vi "RubikStart.vi"() -> (0 "error out":errorcluster)   [LabVIEW 2017, in "RubikLibraryRT.lvlib"]
doc: "Put Rubik's solver into start positions:\nAll servos to 0°, all grippers to closed. \nYou have to position the cube manually!\n\nInput:\n-\n\nOutput:\nError out"
uses:
  RubikLibraryRT.lvlib
  ServoEnumControl.ctl
  ServoAbsAngleControl.ctl
  <vilib>/ErrorRing/Error Ring.xnode
  RubikLibrary.lvlib
panel:
  in  "List of Servo Angles":T1[](array[typedef])=[enum."0°", enum."0°", enum."0°"]
  in  "Gripper closed":bool=TRUE
  in  "List of Servos":T2[](array[typedef])=[enum."Left Servo", enum."Front Servo", enum."Right Servo"]
  # "Rubic Start"
  # "Rubik Cube Start Configuration\n\nPosition of Grippers:  Closed\nPosition of Servos: 0°"
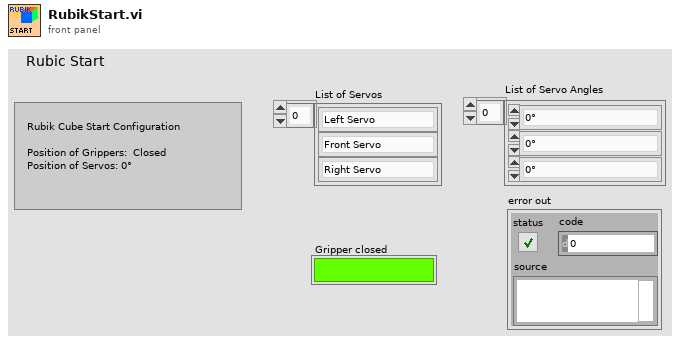
[diagram p1: front panel]
types:
  T1 = typedef "RubikLibrary.lvlib/ServoAbsAngleControl.ctl" = enum16{"+90°", "0°", "-90°"}
  T2 = typedef "RubikLibrary.lvlib/ServoEnumControl.ctl" = enum16{"Left Servo", "Front Servo", "Right Servo"}
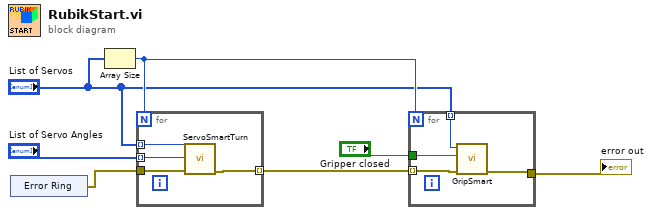
[diagram p0: block diagram]
diagram:
  n1 = xnode "Error Ring"() -> ("error out"=w3:errorcluster)
  n2 = Array Size(array="List of Servos") -> (size(s)=w2:i32)
  n3 = for {
    N: w2 -> [_]
    tunnel: "List of Servos" -> [w11] mode=indexing
    tunnel: "List of Servo Angles" -> [w10] mode=indexing
    tunnel: [w9] -> w5 mode=indexing
    tunnel: w3 -> [w8]
    n4 = call "ServoSmartTurn.vi"("error in"=w8, "Turn to (in)"=w10, "Servo"=w11) -> ("error out"=w9:errorcluster)  [unwired: 7 in, 1 out]
  }
  n5 = for {
    N: w2 -> [_]
    tunnel: [w15] -> w4
    tunnel: "Gripper closed" -> [w14]
    tunnel: "List of Servos" -> [w13] mode=indexing
    tunnel: w5 -> [w12] mode=indexing
    n6 = call "GripSmart.vi"("error in"=w12, "Grip closed (in)"=w14, "Servo"=w13) -> ("error out"=w15:errorcluster)  [unwired: 7 in, 1 out]
  }
  "error out" <- w4
